vi "Initialize Action lists.vi"(7 "Force update list(F)":bool, 11 "error in (no error)":errorcluster) -> (6 "Action names":string[](array[string]), 8 "Actions":T1[](array[typedef]), 15 "error out":errorcluster)   [LabVIEW 2011]
uses:
  Action colleciton cluster.ctl
  Action common elements.ctl
  Action adjuster type.ctl
  Action type.ctl
  General command list.ctl
  PCP interface/High Level/PCP High Level Commands.ctl
  Tool/Stroker/def/Tool specific commands.ctl
  Action cluster Tool.ctl
  Action cluster PCPl.ctl
  Action cluster general.ctl
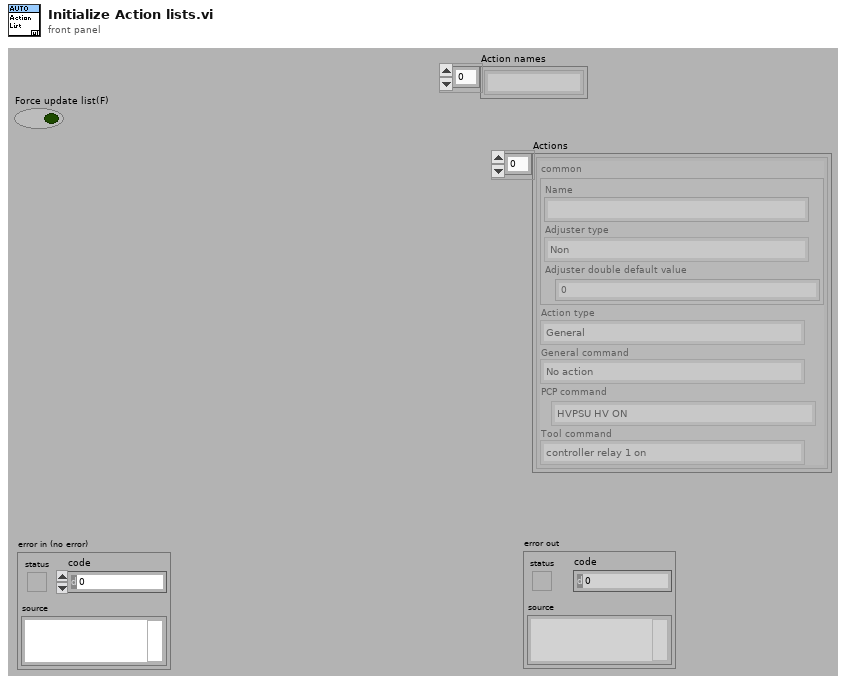
[diagram p1: front panel]
types:
  T1 = typedef "Action colleciton cluster.ctl" = cluster{"common":T2, "Action type":T4, "General command":T5, "PCP command":T6, "Tool command":T7}
  T2 = typedef "Action common elements.ctl" = cluster{"Name":string, "Adjuster type":T3, "Adjuster double default value":dbl}
  T3 = typedef "Action adjuster type.ctl" = enum16{"Non", "Double"}
  T4 = typedef "Action type.ctl" = enum16{"General", "PCP command", "Tool command"}
  T5 = typedef "General command list.ctl" = enum16{"No action"}
  T6 = typedef "PCP High Level Commands.ctl" = enum16{"HVPSU HV ON", "HVPSU HV OFF", "PCP PC", "PCP Local", "Update Motor Voltage", "Update Cable Resistance", "Final Motor Voltage", "Final Resistance"}
  T7 = typedef "Tool specific commands.ctl" = enum16{"controller relay 1 on", "controller relay 1 off", "controller relay 2 on", "controller relay 2 off", "Solonoid 1 (master) on", "Solonoid 1 (master) off", "Solonoid 2 (Stroker) on", "Solonoid 2 (Stroker) off", "Solonoid 3 (Anchor) on", "Solonoid 3 (Anchor) off", "Controller relay 1 & 2 on", "Controller relay 1 & 2 off", "Controller relay 1 on, 2 off", "Controller relay 1 off, 2 on", "STROKER tool: Stop Force Mon", "High-G Stop", "High-G Get data", "High-G Stop Get data", "STROKER tool: Stroke out", "STROKER tool: Stroke in", "STROKER tool: Stroke stop", "STROKER tool: Stroke go to", "STROKER tool: Stop Homing", "STROKER tool: Start Force Mon dir in", "STROKER tool: Start Force Mon dir out", "Controller STOP"}
  T8 = typedef "Action cluster Tool.ctl" = cluster{"common":T2, "Tool command":T7}
  T9 = typedef "Action cluster PCPl.ctl" = cluster{"common":T2, "PCP command":T6}
  T10 = typedef "Action cluster general.ctl" = cluster{"common":T2, "General command":T5}
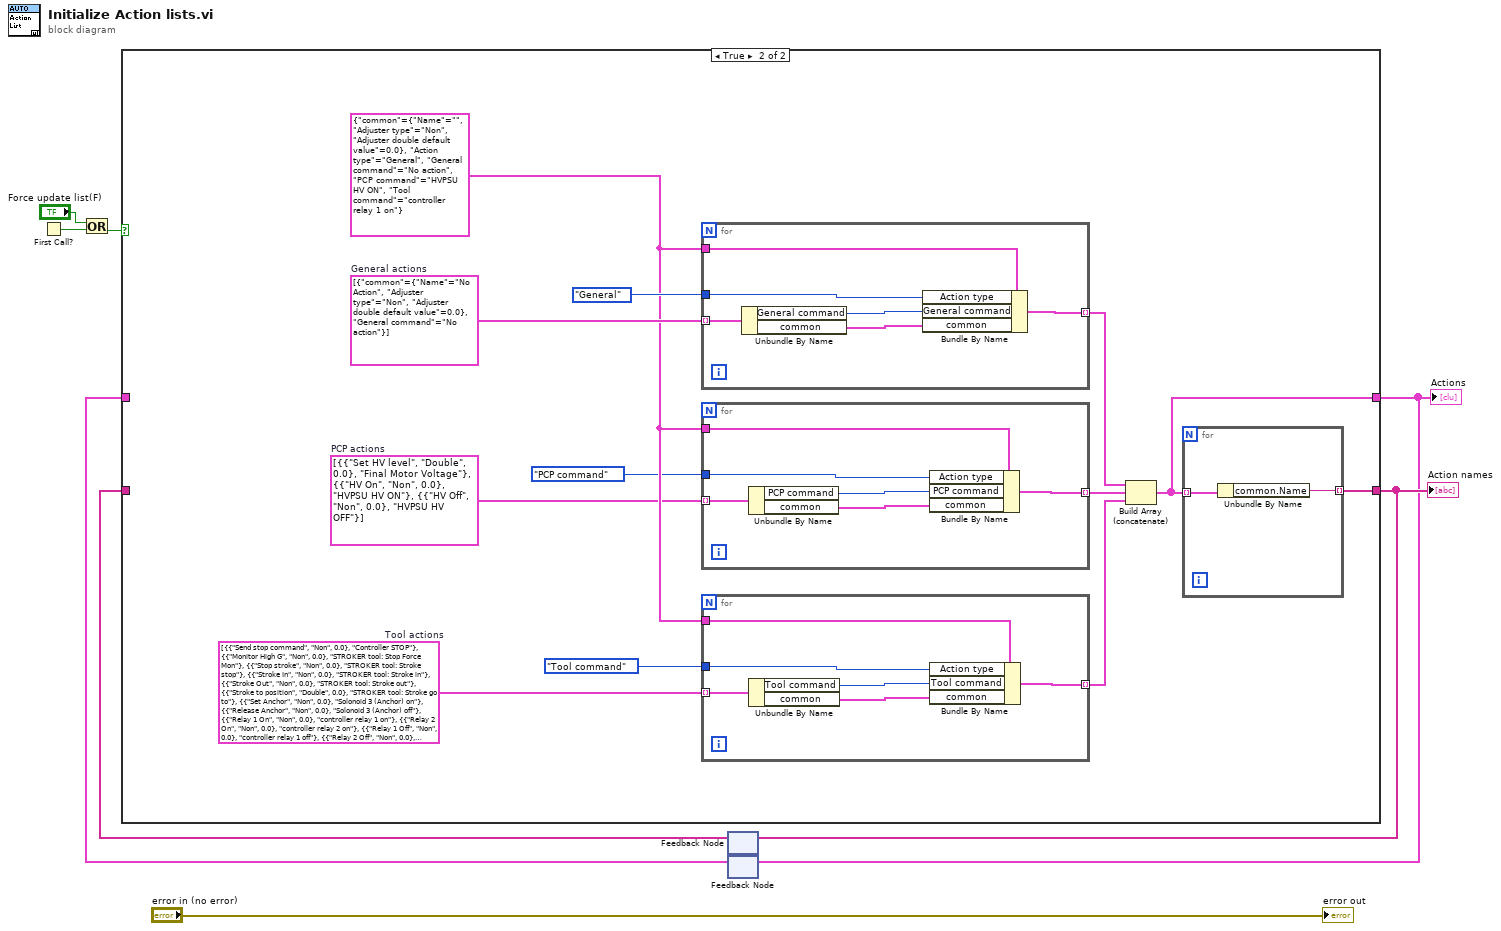
[diagram p0: block diagram]
diagram:
  n1 = First Call?() -> (First Call?: T/F=w8:bool)
  n2 = Or(x="Force update list(F)", y=w8) -> (x .or. y?=w7:bool)
  n3 = feedback #1() -> (w3:string[])  [unwired: 1 in]
  n4 = feedback #2() -> (w2:T1[])  [unwired: 1 in]
  n5 = case shown="True" w7 {
    tunnel: [w9 w12] -> w4
    tunnel: [w10 w11] -> w5
    tunnel: w3 -> [w10 _]
    tunnel: w2 -> [w9 _]
    frame False {
    }
    frame True {
      w20 = T1 {"common"={"Name"="", "Adjuster type"=enum."Non", "Adjuster double default value"=0.0}, "Action type"=enum."General", "General command"=enum."No action", "PCP command"=enum."HVPSU HV ON", "Tool command"=enum."controller relay 1 on"} ("Action")
      w17 = T8[] [{"common"={"Name"="Send stop command", "Adjuster type"=enum."Non", "Adjuster double default value"=0.0}, "Tool command"=enum."Controller STOP"}, {"common"={"Name"="Monitor High G", "Adjuster type"=enum."Non", "Adjuster double default value"=0.0}, "Tool command"=enum."STROKER tool: Stop Force Mon"}, {"common"={"Name"="Stop stroke", "Adjuster type"=enum."Non", "Adjuster double default value"=0.0}, "Tool command"=enum."STROKER tool: Stroke stop"}, {"common"={"Name"="Stroke In", "Adjuster type"=enum."Non", "Adjuster double default value"=0.0}, "Tool command"=enum."STROKER tool: Stroke in"}, {"common"={"Name"="Stroke Out", "Adjuster type"=enum."Non", "Adjuster double default value"=0.0}, "Tool command"=enum."STROKER tool: Stroke out"}, {"common"={"Name"="Stroke to position", "Adjuster type"=enum."Double", "Adjuster double default value"=0.0}, "Tool command"=enum."STROKER tool: Stroke go to"}, {"common"={"Name"="Set Anchor", "Adjuster type"=enum."Non", "Adjuster double default value"=0.0}, "Tool command"=enum."Solonoid 3 (Anchor) on"}, {"common"={"Name"="Release Anchor", "Adjuster type"=enum."Non", "Adjuster double default value"=0.0}, "Tool command"=enum."Solonoid 3 (Anchor) off"}, {"common"={"Name"="Relay 1 On", "Adjuster type"=enum."Non", "Adjuster double default value"=0.0}, "Tool command"=enum."controller relay 1 on"}, {"common"={"Name"="Relay 2 On", "Adjuster type"=enum."Non", "Adjuster double default value"=0.0}, "Tool command"=enum."controller relay 2 on"}, {"common"={"Name"="Relay 1 Off", "Adjuster type"=enum."Non", "Adjuster double default value"=0.0}, "Tool command"=enum."controller relay 1 off"}, {"common"={"Name"="Relay 2 Off", "Adjuster type"=enum."Non", "Adjuster double default value"=0.0}, "Tool command"=enum."controller relay 2 off"}, {"common"={"Name"="Relay 1 and 2 on", "Adjuster type"=enum."Non", "Adjuster double default value"=0.0}, "Tool command"=enum."Controller relay 1 & 2 on"}, {"common"={"Name"="Relay 1 and 2 off", "Adjuster type"=enum."Non", "Adjuster double default value"=0.0}, "Tool command"=enum."Controller relay 1 & 2 off"}, {"common"={"Name"="Relay 1 on,  2 off", "Adjuster type"=enum."Non", "Adjuster double default value"=0.0}, "Tool command"=enum."Controller relay 1 on, 2 off"}, {"common"={"Name"="Relay 1 off,  2 on", "Adjuster type"=enum."Non", "Adjuster double default value"=0.0}, "Tool command"=enum."Controller relay 1 off, 2 on"}, {"common"={"Name"="Start pressure monitoring", "Adjuster type"=enum."Double", "Adjuster double default value"=0.0}, "Tool command"=enum."STROKER tool: Start Force Mon dir in"}, {"common"={"Name"="Stop pressure monitoring", "Adjuster type"=enum."Non", "Adjuster double default value"=0.0}, "Tool command"=enum."STROKER tool: Start Force Mon dir out"}]  # Tool actions
      w19 = T9[] [{"common"={"Name"="Set HV level", "Adjuster type"=enum."Double", "Adjuster double default value"=0.0}, "PCP command"=enum."Final Motor Voltage"}, {"common"={"Name"="HV On", "Adjuster type"=enum."Non", "Adjuster double default value"=0.0}, "PCP command"=enum."HVPSU HV ON"}, {"common"={"Name"="HV Off", "Adjuster type"=enum."Non", "Adjuster double default value"=0.0}, "PCP command"=enum."HVPSU HV OFF"}]  # PCP actions
      w22 = T10[] [{"common"={"Name"="No Action", "Adjuster type"=enum."Non", "Adjuster double default value"=0.0}, "General command"=enum."No action"}]  # General actions
      n6 = for {
        tunnel: w22 -> [w42] mode=indexing
        tunnel: w20 -> [w41]
        tunnel: Action_type."General" ("Action type") -> [w38]
        tunnel: [w37] -> w15 mode=indexing
        n7 = Unbundle By Name(w42) -> ("General command"=w39:T5, "common"=w40:T2)
        n8 = Bundle By Name(cluster=w41, "Action type"=w38, "General command"=w39, "common"=w40) -> (w37:T1)
      }
      n9 = for {
        tunnel: w19 -> [w36] mode=indexing
        tunnel: w20 -> [w35]
        tunnel: Action_type."PCP command" ("Action type") -> [w32]
        tunnel: [w31] -> w14 mode=indexing
        n10 = Unbundle By Name(w36) -> ("PCP command"=w33:T6, "common"=w34:T2)
        n11 = Bundle By Name(cluster=w35, "Action type"=w32, "PCP command"=w33, "common"=w34) -> (w31:T1)
      }
      n12 = for {
        tunnel: w17 -> [w30] mode=indexing
        tunnel: w20 -> [w29]
        tunnel: Action_type."Tool command" ("Action type") -> [w26]
        tunnel: [w25] -> w13 mode=indexing
        n13 = Unbundle By Name(w30) -> ("Tool command"=w27:T7, "common"=w28:T2)
        n14 = Bundle By Name(cluster=w29, "Action type"=w26, "Tool command"=w27, "common"=w28) -> (w25:T1)
      }
      n15 = Build Array (concatenate)(w15, w14, w13) -> (w12:T1[])
      n16 = for {
        tunnel: w12 -> [w24] mode=indexing
        tunnel: [w23] -> w11 mode=indexing
        n17 = Unbundle By Name(w24) -> ("common.Name"=w23:string)
      }
    }
  }
  "Actions" <- w4
  "Action names" <- w5
  n18 = feedback-in #1(w5) -> ()
  n19 = feedback-in #2(w4) -> ()
  "error out" <- "error in (no error)"
